vi "dfd_Get Frequency Points (Log-Spaced).vi"(10 "order":i32, 11 "plot settings":T1={"# freq bins"=-1, "low frequency [Hz]"=0.01, "high frequency [Hz]"=0.5}) -> (3 "freq points":dbl[](array[numeric]) format="%#_40g")   [LabVIEW 2017, in "NI_DigFilterLicensed.lvlib"]
uses:
  <vilib>/addons/Digital Filter Design/NI_DigFilterLicensed.lvlib
  <vilib>/addons/Digital Filter Design/_Objects.llb/DFD Plot Settings.ctl
  <vilib>/Analysis/1siggen.llb/Ramp Pattern by Samples.vi
  <vilib>/Analysis/NI_AALBase.lvlib
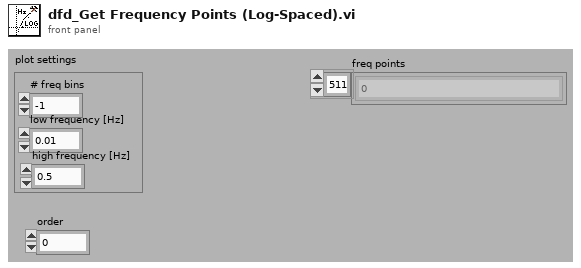
[diagram p1: front panel]
types:
  T1 = typedef "NI_DigFilterLicensed.lvlib/DFD Plot Settings.ctl" = cluster{"# freq bins":i32, "low frequency [Hz]":dbl, "high frequency [Hz]":dbl}
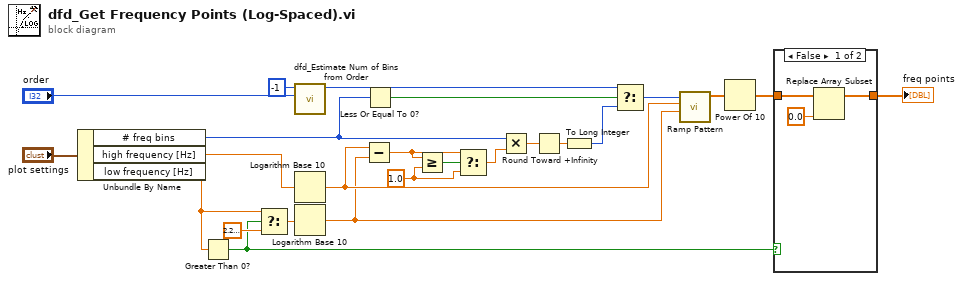
[diagram p0: block diagram]
diagram:
  w7 = 1.0 ("y")
  n1 = Unbundle By Name("plot settings") -> ("# freq bins"=w18:i32, "high frequency [Hz]"=w20:dbl, "low frequency [Hz]"=w4:dbl)
  n2 = Greater Than 0?(x=w4) -> (x > 0?=w1:bool)
  n3 = Select(t=w4, s=w1, f=2.220446049250313e-16) -> (s? t:f=w5:dbl)
  n4 = call <vilib>:"dfd_Estimate Num of Bins from Order.vi"("order"="order", "# freq bins in"=-1) -> ("# freq bins out"=w19:i32)  [unwired: 9 in]
  n5 = Logarithm Base 10(1:w20) -> (0:w11:dbl)
  n6 = Logarithm Base 10(1:w5) -> (0:w10:dbl)
  n7 = Subtract(x=w11, y=w10) -> (x-y=w8:dbl)
  n8 = Less Or Equal To 0?(x=w18) -> (x <= 0?=w22:bool)
  n9 = Greater Or Equal?(x=w8, y=w7) -> (x >= y?=w9:bool)
  n10 = Select(t=w8, s=w9, f=w7) -> (s? t:f=w6:dbl)
  n11 = Multiply(x=w18, y=w6) -> (x*y=w17:dbl)
  n12 = Round Toward +Infinity(x=w17) -> (ceil(x): smallest int >= x=w16:dbl)
  n13 = To Long Integer(number=w16) -> (32bit integer=w15:i32)
  n14 = Select(t=w19, s=w22, f=w15) -> (s? t:f=w12:i32)
  n15 = call-poly <vilib>:"Ramp Pattern.vi"("start"=w10, "end"=w11, "samples"=w12) -> ("Ramp Pattern"=w23:dbl[])  [unwired: 7 in, 1 out]
  n16 = Power Of 10(x=w23) -> (10^x=w24:dbl[])
  n17 = case shown="False" w1 {
    tunnel: w24 -> [w27 w28]
    tunnel: [w26 w28] -> w2
    frame False {
      n18 = Replace Array Subset(array=w27, new element=0.0 ("new element/subarray")) -> (w26:dbl[])  [unwired: 1 in]
    }
    frame True {
    }
  }
  "freq points" <- w2
